vi "onProcessStarted.vi"(8 "error in (no error)":errorcluster, 11 "MAUI":refnum<class "MAUI.lvclass">) -> (0 "error out":errorcluster, 3 "MAUI out":refnum<class "MAUI.lvclass">)   [LabVIEW 2019, in "MAUI.lvclass"]
doc: "JKI State Machine Objects (SMO) 1.3.0.56\nJKI - JKI\nCopyright (c) 2017, JKI"
uses:
  MAUI.lvclass
  <vilib>/JKI/JKI SMO/SMO.UI/SMO.UI.lvclass
  <vilib>/JKI/JKI SMO/SMO/SMO.lvclass
  <userlib>/LevyLab/Embedded UI/Embedded UI/Embedded UI.lvclass
  C:/Program Files (x86)/National Instruments/LabVIEW 2019/vi.lib/JKI/JKI SMO/SMO/SMO.lvclass
panel:
  # "For instructions on how to use the JKI State Machine Objects, examples and video tutorials, visit:\nhttp://jki.net/state-machine-objects/\n\nJKI State Machine Objects™\nhttp://jki.net/state-machine-objects/\nCopyright (C) 2005-2015, JKI <info@jki.net>\nALL RIGHTS RESERVED"
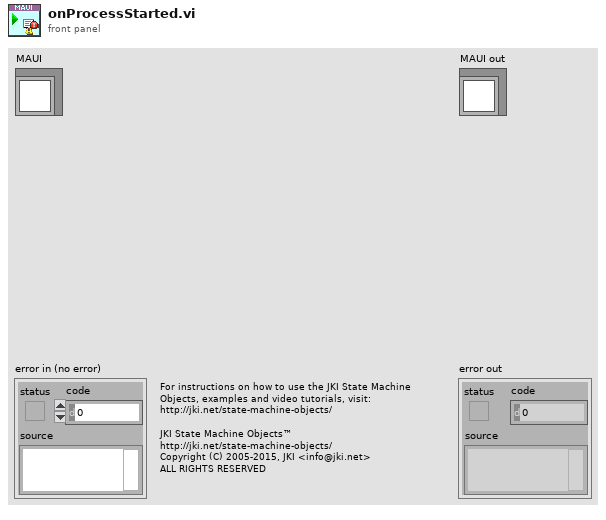
[diagram p1: front panel]
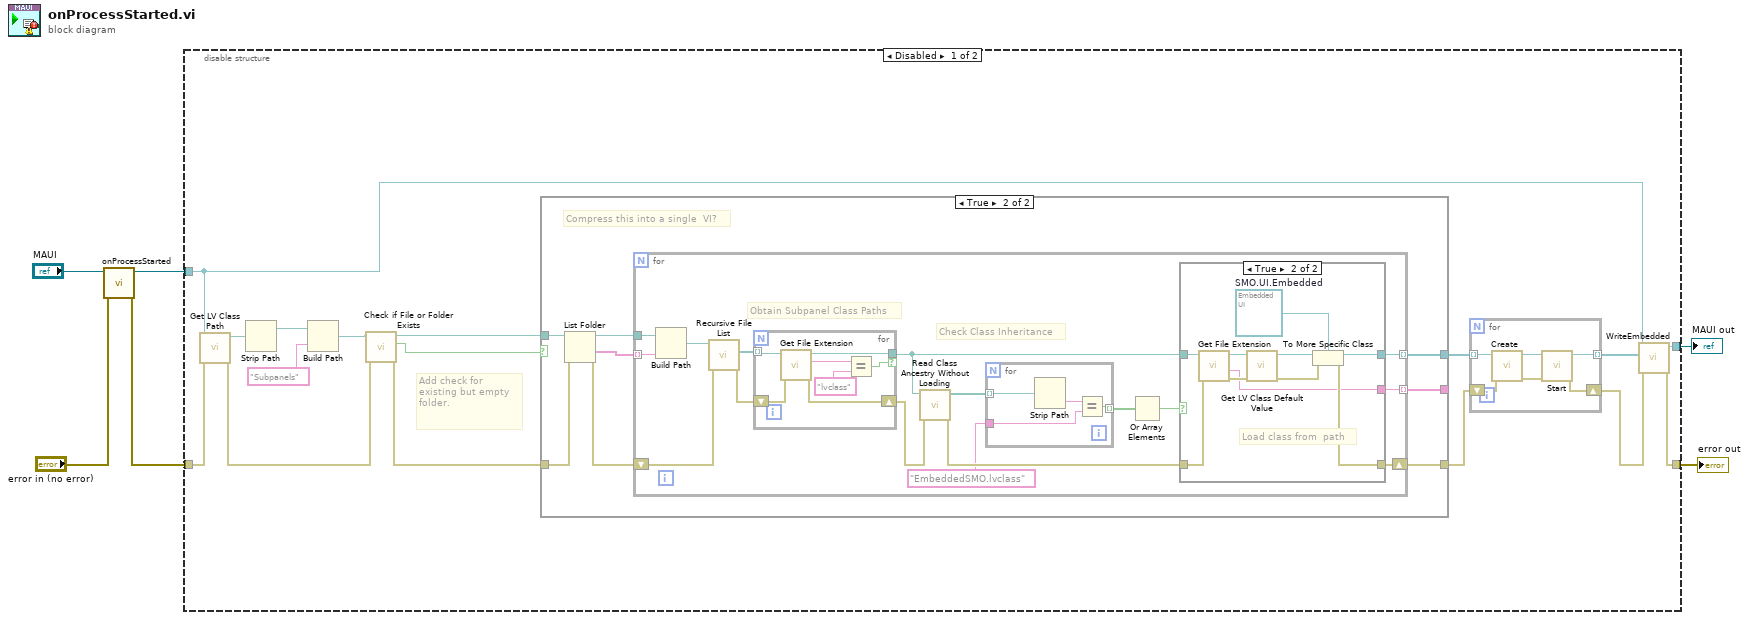
[diagram p0: block diagram]
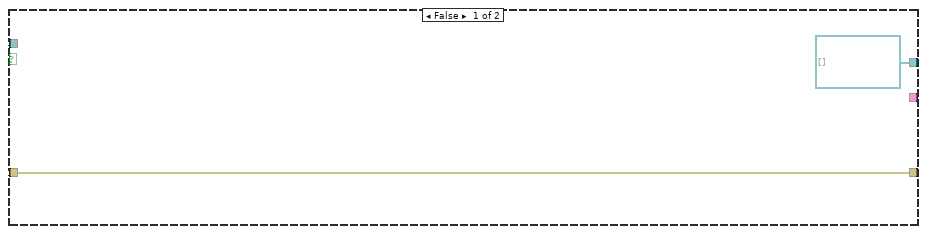
[diagram p2: hidden frame]
diagram:
  n1 = call-parent "onProcessStarted.vi"("error in (no error)"="error in (no error)", "SMO"="MAUI") -> ("error out"=w5:errorcluster, "SMO out"=w2:refnum<class "MAUI.lvclass">)  [unwired: 8 in]
  n2 = disable-structure shown="Disabled" {
    disable-tunnel: w5 -> [w20 w79]
    disable-tunnel: w2 -> [w10 w78]
    disable-tunnel: [w19 w79] -> w4
    disable-tunnel: [w9 w78] -> w1
    frame Disabled {
      # "Add check for existing but empty folder."
      n3 = call <vilib>:"Get LV Class Path.vi"("error in (no error)"=w20, "object"=w10) -> ("error out"=w21:errorcluster, "class path"=w16:path)  [unwired: 8 in]
      n4 = Strip Path(path=w16) -> (stripped path=w15:path)  [unwired: 1 out]
      n5 = Build Path(base path=w15, name or relative path="Subpanels") -> (appended path=w13:path)
      n6 = call <vilib>:"Check if File or Folder Exists.vi"("error in (no error)"=w21, "path"=w13) -> ("error out"=w22:errorcluster, "file or folder exists?"=w11:bool, "dup path"=w12:path)  [unwired: 7 in]
      n7 = case shown="True" w11 {
        tunnel: w12 -> [w30 w36]
        tunnel: w22 -> [w31 w38]
        tunnel: [w31 w37] -> w17
        tunnel: [refnum<class "Embedded UI.lvclass">[] [] w33] -> w8
        tunnel: [_ w32] -> _
        frame False {
          n8 = Create Folder(path (use dialog)=w30, error in=w31) -> ()  [unwired: 1 in, 3 out]
        }
        frame True {
          # "Compress this into a single  VI?"
          n9 = List Folder(path=w36, error in=w38) -> (path out=w35:path, folder names=w34:string[], error out=w39:errorcluster)  [unwired: 2 in, 1 out]
          n10 = for {
            tunnel: w35 -> [w50]
            tunnel: w34 -> [w49] mode=indexing
            tunnel: [w45] -> w33 mode=indexing
            shift-right: [w51] -> w37
            shift-left: w39 -> [w55]
            tunnel: [w40] -> w32 mode=indexing
            # "Check Class Inheritance"
            # "Obtain Subpanel Class Paths"
            n11 = Build Path(base path=w50, name or relative path=w49) -> (appended path=w48:path)
            n12 = call <vilib>:"Recursive File List.vi"("error in (no error)"=w55, "Folder Path"=w48) -> ("error out"=w54:errorcluster, "All Files in Dir"=w47:path[])  [unwired: 5 in, 3 out]
            n13 = for {
              tunnel: w47 -> [w73] mode=indexing
              tunnel: [w72] -> w46 if=w71
              shift-right: [w76] -> w53
              shift-left: w54 -> [w77]
              n14 = call <vilib>:"Get File Extension.vi"("error in (no error)"=w77, "file"=w73) -> ("error out"=w76:errorcluster, "lowercase file extension"=w75:string, "dup file"=w72:path)  [unwired: 5 in, 2 out]
              n15 = Equal?(x=w75, y="lvclass") -> (x = y?=w71:bool)
            }
            n16 = call <vilib>:"Read Class Ancestry Without Loading.vi"("error in (no error)"=w53, "LabVIEW Class Path"=w46) -> ("error out"=w52:errorcluster, "Class Ancestry"=w44:path[])  [unwired: 8 in]
            n17 = for {
              tunnel: w44 -> [w70] mode=indexing
              tunnel: [w68] -> w43 mode=indexing
              tunnel: "EmbeddedSMO.lvclass" -> [w67]
              n18 = Strip Path(path=w70) -> (name=w69:string)  [unwired: 1 out]
              n19 = Equal?(x=w69, y=w67) -> (x = y?=w68:bool)
            }
            n20 = Or Array Elements(Boolean array=w43) -> (logical OR=w41:bool)
            n21 = case shown="True" w41 {
              tunnel: w46 -> [_ w60]
              tunnel: [_ w62] -> w45
              tunnel: w52 -> [w56 w64]
              tunnel: [w56 w65] -> w51
              tunnel: [_ w58] -> w40
              frame False {
              }
              frame True {
                w57 = refnum<class "Embedded UI.lvclass"> refnum  # SMO.UI.Embedded
                # "Load class from  path"
                n22 = call <vilib>:"Get File Extension.vi"("error in (no error)"=w64, "file"=w60) -> ("error out"=w63:errorcluster, "filename without extension"=w58:string, "dup file"=w59:path)  [unwired: 5 in, 2 out]
                n23 = call <vilib>:"Get LV Class Default Value.vi"("error in (no error)"=w63, "class path"=w59) -> ("error out"=w66:errorcluster, "object"=w61:refnum<class>)  [unwired: 8 in]
                n24 = To More Specific Class(target class=w57, reference=w61, error in=w66) -> (specific class reference=w62:refnum<class "Embedded UI.lvclass">, error out=w65:errorcluster)
              }
            }
          }
        }
      }
      n25 = for {
        tunnel: w8 -> [w25] mode=indexing
        tunnel: [w24] -> w7 mode=indexing
        shift-right: [w26] -> w18
        shift-left: w17 -> [w27]
        n26 = call <vilib>:"Create.vi"("error in (no error)"=w27, "SMO"=w25) -> ("error out"=w28:errorcluster, "SMO out"=w23:refnum<class "Embedded UI.lvclass">)  [unwired: 7 in, 1 out]
        n27 = call <vilib>:"Start.vi"("error in (no error)"=w28, "SMO"=w23) -> ("error out"=w26:errorcluster, "SMO out"=w24:refnum<class "Embedded UI.lvclass">)  [unwired: 8 in]
      }
      n28 = call "WriteEmbedded.vi"("error in (no error)"=w18, "Subpanels"=w7, "MAUI in"=w10) -> ("error out"=w19:errorcluster, "MAUI out"=w9:refnum<class "MAUI.lvclass">)  [unwired: 7 in]
    }
    frame Enabled {
    }
  }
  "error out" <- w4
  "MAUI out" <- w1
